vi "potential-field.vi"(11 "IA State Output in":T1={"our_robots"=[], "enemy_robots"=[], "balls"=[], "geometry"={"line_width"=0, "field_length"=0, "field_width"=0, "boundary_width"=0, "referee_width"=0, "goal_width"=0, "goal_depth"=0, "goal_wall_width"=0, "center_circle_radius"=0, "defense_radius"=0, "defense_stretch"=0, "free_kick_from_defense_dist"=0, "penalty_spot_from_field_line_dist"=0, "penalty_line_from_spot_dist"=0}, "IA Judge"={"stage"="", "command"="", "our_goalie_id"=0.0, "enemy_goalie_id"=0.0, "command enum"=enum."Halt", "Time"=enum."Azul"}, "Received Timestamp"=timestamp(0 s since 1904-01-01), "Events"={"Touch"=FALSE, "Ball out"=FALSE, "id touch"=0.0, "Ball out of \nVision"=FALSE, "Ball inside \nGoalie area"=FALSE, "Robot not responding"=FALSE, "Robots responding status"=[1.0, 1.0, 1.0, 1.0, 1.0, 1.0], "Enemy Ball \nPossession"=FALSE, "Pass State"=FALSE, "id end of pass"=0.0, "Kick"=FALSE, "Id ini Possession"=0.0, "Ball Possesion"=FALSE, "Id Possesion"=0.0, "Direct Kick"=FALSE, "2nd Strk Ativo"=FALSE}}) -> (3 "IA State Output out":T1={"our_robots"=[], "enemy_robots"=[], "balls"=[], "geometry"={"line_width"=0, "field_length"=0, "field_width"=0, "boundary_width"=0, "referee_width"=0, "goal_width"=0, "goal_depth"=0, "goal_wall_width"=0, "center_circle_radius"=0, "defense_radius"=0, "defense_stretch"=0, "free_kick_from_defense_dist"=0, "penalty_spot_from_field_line_dist"=0, "penalty_line_from_spot_dist"=0}, "IA Judge"={"stage"="", "command"="", "our_goalie_id"=0.0, "enemy_goalie_id"=0.0, "command enum"=enum."Halt", "Time"=enum."Azul"}, "Received Timestamp"=timestamp(0 s since 1904-01-01), "Events"={"Touch"=FALSE, "Ball out"=FALSE, "id touch"=0.0, "Ball out of \nVision"=FALSE, "Ball inside \nGoalie area"=FALSE, "Robot not responding"=FALSE, "Robots responding status"=[1.0, 1.0, 1.0, 1.0, 1.0, 1.0], "Enemy Ball \nPossession"=FALSE, "Pass State"=FALSE, "id end of pass"=0.0, "Kick"=FALSE, "Id ini Possession"=0.0, "Ball Possesion"=FALSE, "Id Possesion"=0.0, "Direct Kick"=FALSE, "2nd Strk Ativo"=FALSE}})   [LabVIEW 2018]
uses:
  Communication_class/Paths/MessageAI_State Folder/Core/AI Input.ctl
  Vision_class/Old vision/Controls/AI Robot.ctl
  Vision_class/Old vision/Controls/Functions Enum.ctl
  Vision_class/Old vision/Controls/AttackerStates.ctl
  Vision_class/Old vision/Controls/PathDests.ctl
  Vision_class/Old vision/Controls/PathDest.ctl
  Communication_class/Paths/MessageAI_State Folder/Core/AI Ball.ctl
  Communication_class/Paths/MessageAI_State Folder/Core/Field Size.ctl
  Communication_class/Paths/MessageAI_State Folder/Core/AI Judge.ctl
  Communication_class/Paths/MessageAI_State Folder/Intel/Command Enum.ctl
  Communication_class/Paths/MessageAI_State Folder/Util/Events/Events.ctl
  <vilib>/Analysis/_algsub.llb/Vector Norm Type.ctl
  <vilib>/Analysis/_algsub.llb/Real Vector Norm.vi
  <vilib>/Analysis/coordinate.llb/2D Cartesian Coordinate Rotation (Scalar).vi
  <vilib>/Analysis/NI_AALPro.lvlib
panel:
  in  "influence radius":dbl=500.0 format="%#_13g"
  in  "multiplier":dbl(slide)=1.0 scale=0.0..10.0
  in  "dist to nullify pot field":dbl=800.0 format="%#_13g"
  in  "min dist to reduce":dbl=500.0 format="%#_13g"
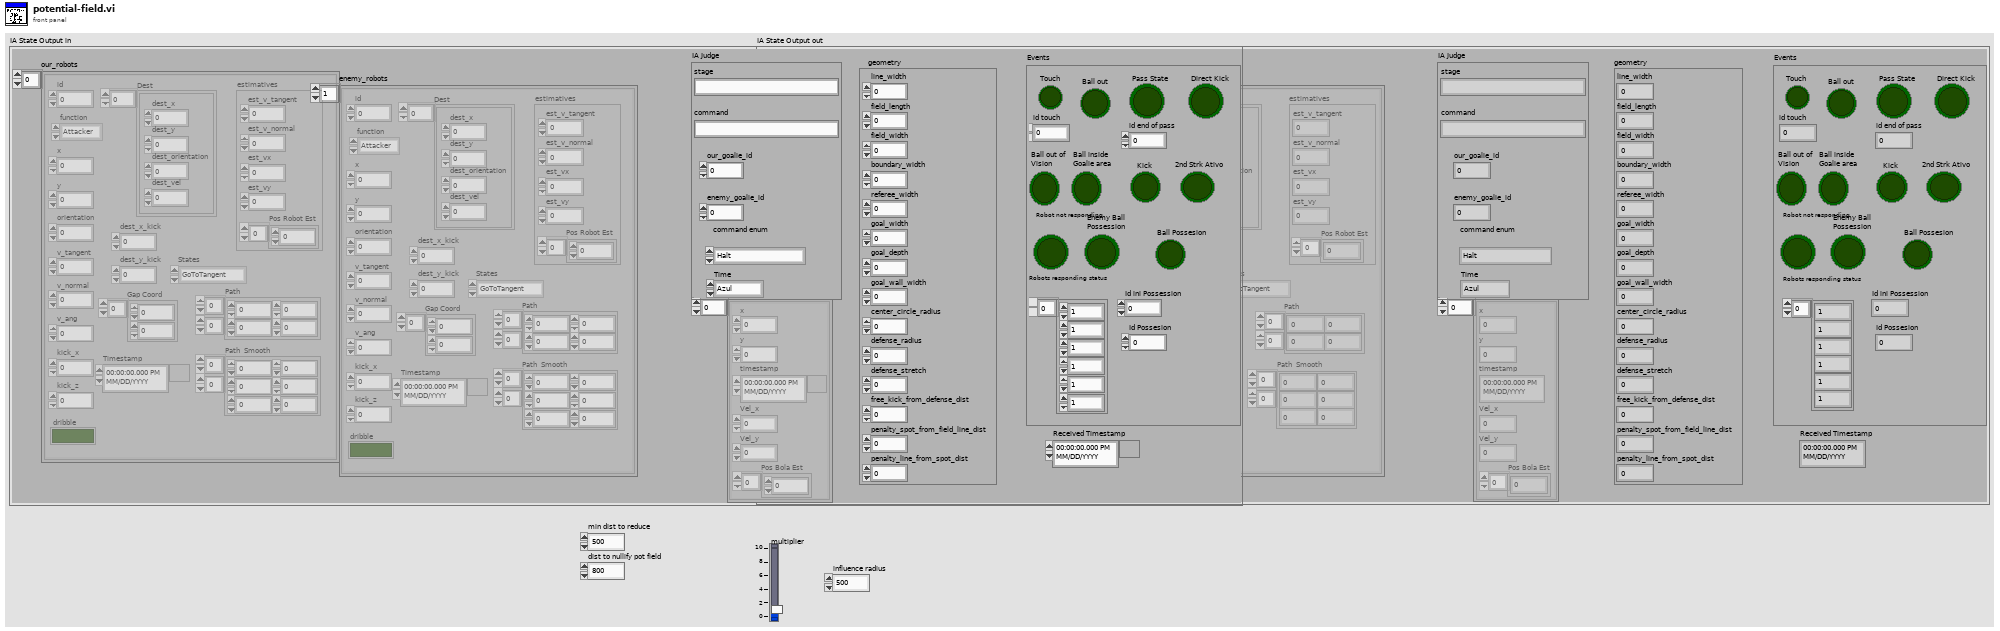
[diagram p1: front panel]
types:
  T1 = typedef "AI Input.ctl" = cluster{"our_robots":T2[], "enemy_robots":T2[], "balls":T7[], "geometry":T8, "IA Judge":T9, "Received Timestamp":timestamp, "Events":T11}
  T2 = typedef "AI Robot.ctl" = cluster{"id":u32, "function":T3, "x":dbl, "y":dbl, "orientation":dbl, "v_tangent":dbl, "v_normal":dbl, "v_ang":dbl, "kick_x":dbl, "kick_z":dbl, "dribble":bool, "Timestamp":timestamp, "estimatives":cluster{"est_v_tangent":dbl, "est_v_normal":dbl, "est_vx":dbl, "est_vy":dbl, "Pos Robot Est":dbl[]}, "dest_x_kick":dbl, "dest_y_kick":dbl, "Gap Coord":dbl[], "States":T4, "Path ":dbl[][], "Path  Smooth":dbl[][], "Dest":T5}
  T3 = typedef "Functions Enum.ctl" = enum16{"2nd Striker", "Attacker", "Goalie", "Defender", "Striker", "Goto 0", "Dummy", "Kicker", "ZigZag 0", "ZigZag 1", "ZigZag 2", "ZigZag 3", "ZigZag 4", "ZigZag 5", "ZigZag 6", "ZigZag 7", "ZigZag 8", ""}
  T4 = typedef "AttackerStates.ctl" = enum16{"Pass", "GoToTangent", "BallGetting", "GoToKick", ""}
  T5 = typedef "PathDests.ctl" = T6[]
  T6 = typedef "PathDest.ctl" = cluster{"dest_x":dbl, "dest_y":dbl, "dest_orientation":dbl, "dest_vel":dbl}
  T7 = typedef "AI Ball.ctl" = cluster{"x":dbl, "y":dbl, "timestamp":timestamp, "Vel_x":dbl, "Vel_y":dbl, "Pos Bola Est":dbl[]}
  T8 = typedef "Field Size.ctl" = cluster{"line_width":u32, "field_length":u32, "field_width":u32, "boundary_width":u32, "referee_width":u32, "goal_width":u32, "goal_depth":u32, "goal_wall_width":u32, "center_circle_radius":u32, "defense_radius":u32, "defense_stretch":u32, "free_kick_from_defense_dist":u32, "penalty_spot_from_field_line_dist":u32, "penalty_line_from_spot_dist":u32}
  T9 = typedef "AI Judge.ctl" = cluster{"stage":string, "command":string, "our_goalie_id":dbl, "enemy_goalie_id":dbl, "command enum":T10, "Time":enum16{"Azul", "Amarelo"}}
  T10 = typedef "Command Enum.ctl" = enum16{"Halt", "Stop", "Force Start", "PKA Normal Start", "Prepare Kickoff Ally", "PKE Normal Start", "Prepare Kickoff Enemy", "Prepare Penalty Ally", "PPA Normal Start", "Prepare Penalty Enemy", "PPE Normal Start", "Direct Free Enemy", "Direct Free Ally", "Indirect Free Enemy", "Indirect Free Ally", "Timeout Enemy", "Timeout Ally", "Goal Enemy", "Goal Ally", "Ball Placement Enemy", "Ball Placement Ally", "Normal Half Time", "Extra Time Break", "Extra Half Time", "None", "Post Game"}
  T11 = typedef "Events.ctl" = cluster{"Touch":bool, "Ball out":bool, "id touch":dbl, "Ball out of \nVision":bool, "Ball inside \nGoalie area":bool, "Robot not responding":bool, "Robots responding status":dbl[], "Enemy Ball \nPossession":bool, "Pass State":bool, "id end of pass":dbl, "Kick":bool, "Id ini Possession":dbl, "Ball Possesion":bool, "Id Possesion":dbl, "Direct Kick":bool, "2nd Strk Ativo":bool}
  T12 = typedef "NI_AALPro.lvlib/Vector Norm Type.ctl" = u16
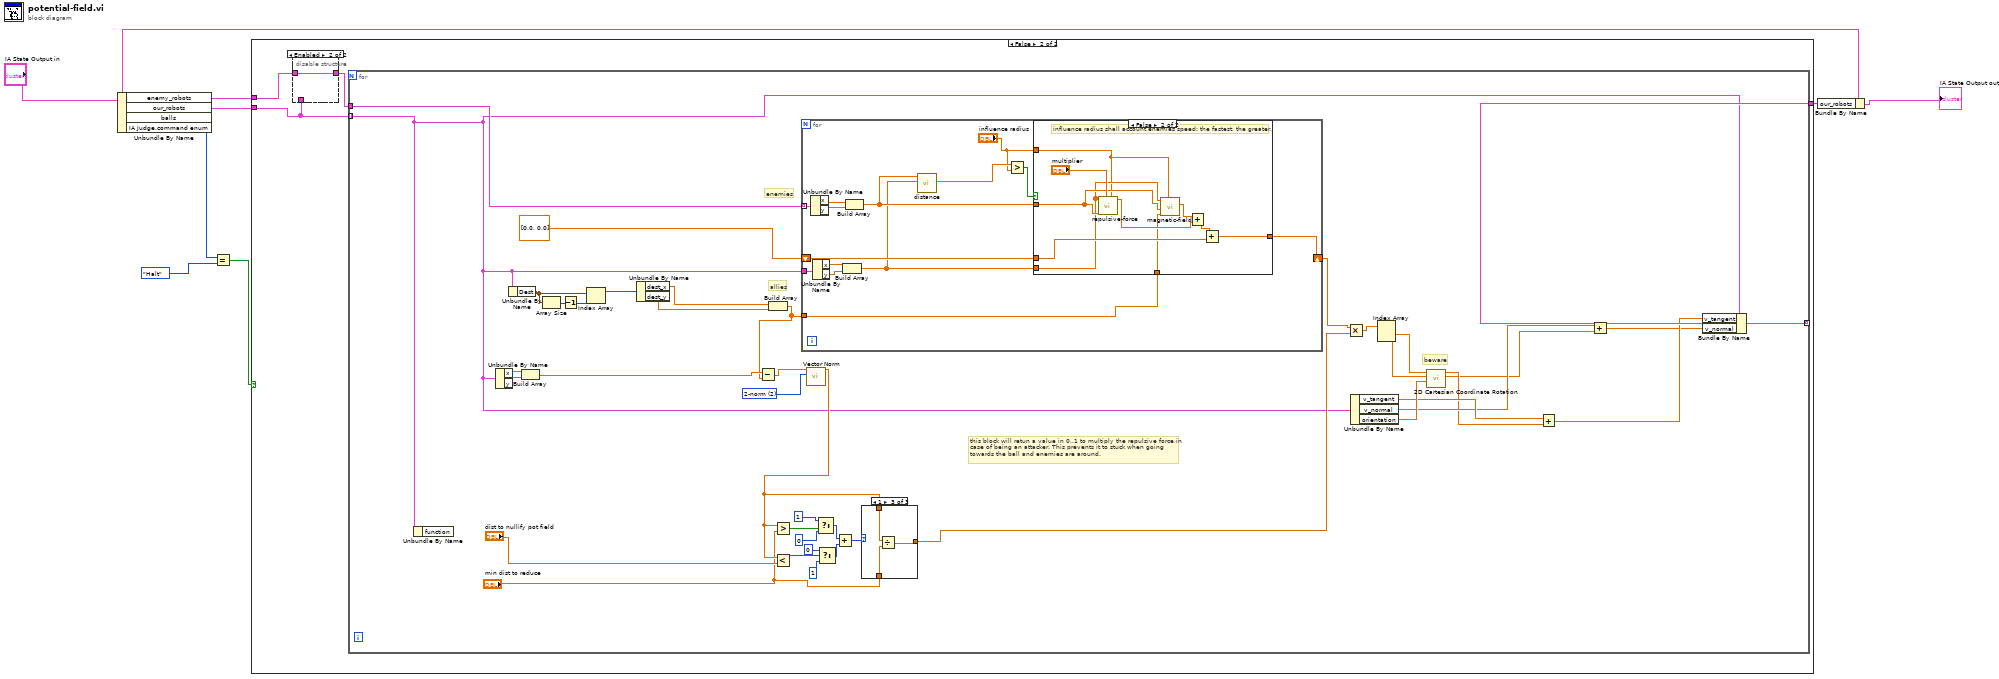
[diagram p0: block diagram]
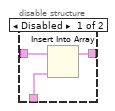
[diagram p3: hidden frame]
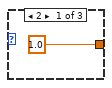
[diagram p4: hidden frame]
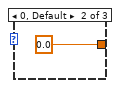
[diagram p5: hidden frame]
diagram:
  n1 = Unbundle By Name("IA State Output in") -> ("enemy_robots"=w8:T2[], "our_robots"=w7:T2[], "IA Judge.command enum"=w3:T10)  [unwired: 1 out]
  n2 = Equal?(x=w3, y=Command_Enum."Halt") -> (x = y?=w1:bool)
  n3 = case shown="False" w1 {
    tunnel: w8 -> [_ w12]
    tunnel: w7 -> [w9 w11]
    tunnel: [w9 w13] -> w6
    frame True {
    }
    frame False {
      n4 = disable-structure shown="Enabled" {
        disable-tunnel: w12 -> [w16 w17]
        disable-tunnel: w11 -> [w15 _]
        disable-tunnel: [w14 w17] -> w10
        frame Disabled {
          n5 = Insert Into Array(array=w16, new element=w15) -> (w14:T2[])  [unwired: 1 in]
        }
        frame Enabled {
        }
      }
      n6 = for {
        tunnel: w10 -> [w57]
        tunnel: w11 -> [w36] mode=indexing
        tunnel: [w47] -> w13 mode=indexing
        w38 = T12 2 items=["1-norm"=1, "2-norm"=2, "Inf-norm"=3, "-Inf-norm"=4, "User Defined"=5] ("norm type")
        # "allies"
        # "enemies"
        # "this block will retun a value in 0..1 to multiply the repulsive force in\ncase of being an attacker. This prevents it to stuck when going \ntowards the ball and enemies are around."
        # "beware"
        n7 = Unbundle By Name(w36) -> ()  [unwired: 1 out]
        n8 = Unbundle By Name(w36) -> ("x"=w42:dbl, "y"=w41:dbl)
        n9 = Unbundle By Name(w36) -> ("Dest"=w20:T5)
        n10 = Build Array(w42, w41) -> (w40:dbl[])
        n11 = Array Size(array=w20) -> (size(s)=w23:i32)
        n12 = Decrement(x=w23) -> (x-1=w22:i32)
        n13 = Index Array(array=w20, index=w22) -> (element=w21:T6)
        n14 = Unbundle By Name(w21) -> ("dest_x"=w19:dbl, "dest_y"=w18:dbl)
        n15 = Build Array(w19, w18) -> (w35:dbl[])
        n16 = Subtract(x=w40, y=w35) -> (x-y=w39:dbl[])
        n17 = for {
          tunnel: w57 -> [w76] mode=indexing
          tunnel: w36 -> [w69]
          shift-right: [w70] -> w45
          shift-left: dbl[] [0.0, 0.0] -> [w71]
          tunnel: w35 -> [w66]
          n18 = Unbundle By Name(w76) -> ("x"=w75:dbl, "y"=w74:dbl)
          n19 = Unbundle By Name(w69) -> ("x"=w73:dbl, "y"=w72:dbl)
          n20 = Build Array(w73, w72) -> (w67:dbl[])
          n21 = Build Array(w75, w74) -> (w68:dbl[])
          n22 = call "distance.vi"("P1"=w67, "P2"=w68) -> ("Dist P1P2"=w65:dbl)  [unwired: 9 in]
          n23 = Greater?(x=w65, y="influence radius") -> (0:w63:bool)
          n24 = case shown="False" w63 {
            tunnel: w71 -> [w77 w87]
            tunnel: [w77 w86] -> w70
            tunnel: w68 -> [_ w81]
            tunnel: w67 -> [_ w80]
            tunnel: w66 -> [_ w79]
            tunnel: "influence radius" -> [_ w78]
            frame True {
            }
            frame False {
              # "influence radius shall account enemies speed: the fastest, the greater."
              n25 = call "repulsive-force.vi"("influence radius"=w78, "multiplier"="multiplier", "obstacle pos"=w81, "agent pos"=w80) -> ("force"=w84:dbl[])  [unwired: 6 in, 1 out]
              n26 = call "magnetic-field.vi"("enemy influence radius"=w78, "goal pos"=w79, "enemy pos"=w81, "ally pos"=w80) -> ("magnetic force"=w85:dbl[])  [unwired: 7 in]
              n27 = Add(x=w85, y=w84) -> (x+y=w83:dbl[])
              n28 = Add(x=w83, y=w87) -> (x+y=w86:dbl[])
            }
          }
        }
        n29 = call-poly <vilib>:"Vector Norm.vi"("norm type"=w38, "Input Vector"=w39) -> ("norm"=w37:dbl)  [unwired: 8 in, 1 out]
        n30 = Less?(x=w37, y="dist to nullify pot field") -> (x < y?=w31:bool)
        n31 = Greater?(x=w37, y="min dist to reduce") -> (0:w32:bool)
        n32 = Select(t=1, s=w32, f=0) -> (s? t:f=w33:i32)
        n33 = Select(t=0, s=w31, f=1) -> (s? t:f=w34:i32)
        n34 = Add(x=w33, y=w34) -> (x+y=w25:i32)
        n35 = case shown="1" w25 {
          tunnel: [1.0 0.0 w60] -> w44
          tunnel: w37 -> [_ _ w62]
          tunnel: "min dist to reduce" -> [_ _ w61]
          frame 2 {
          }
          frame 0, Default {
          }
          frame 1 {
            n36 = Divide(x=w62, y=w61) -> (x/y=w60:dbl)
          }
        }
        n37 = Multiply(x=w45, y=w44) -> (x*y=w43:dbl[])
        n38 = Unbundle By Name(w36) -> ("v_tangent"=w53:dbl, "v_normal"=w52:dbl, "orientation"=w54:dbl)
        n39 = Index Array(array=w43) -> (element #1=w56:dbl, element #2=w55:dbl)  [unwired: 2 in]
        n40 = call-poly <vilib>:"2D Cartesian Coordinate Rotation.vi"("theta"=w54, "y"=w55, "x"=w56) -> ("y out"=w50:dbl, "x out"=w51:dbl)  [unwired: 6 in, 1 out]
        n41 = Add(x=w53, y=w51) -> (x+y=w49:dbl)
        n42 = Add(x=w52, y=w50) -> (x+y=w48:dbl)
        n43 = Bundle By Name(cluster=w36, "v_tangent"=w49, "v_normal"=w48) -> (w47:T2)
      }
    }
  }
  n44 = Bundle By Name(cluster="IA State Output in", "our_robots"=w6) -> (→"IA State Output out":T1)
